vi "test_asap_coupling.vi"() -> ()   [LabVIEW 2013]
uses:
  <vilib>/Analysis/Matrix/Datatypes/RealMatrix.ctl
  <vilib>/Analysis/6fits.llb/Curve Fitting Criteria.ctl
  initialization/micron_globals.vi
  <vilib>/Analysis/Matrix/Numeric/Conversions/Array To Matrix - RA.vi
  <vilib>/Analysis/Matrix/NI_Matrix.lvlib
  <vilib>/Analysis/NI_AALPro.lvlib
panel:
  out "slope":dbl format="%#_3p"
  in  "Fit method":T1=2 items=["Least Square", "Least Absolute Residual", "Bisquare"]
  out "Error vs. sensor plane distance":cluster{cluster{sgl, "Numeric":dbl}[]}[](graph)
  out "Two-on error (axis sum, normalized)":T2 format="%#_3p"
  out "Sensor 1 1/dist":T2 format="%#_3p"
  out "Sensor 0 1/dist":T2 format="%#_3p"
  out "All-on sum":T2 format="%#_3p"
  out "Two-on error (axis sum, um)":T2 format="%#_3p"
  out "All-on axis error (um)":T2 format="%#_3p"
  out "Coupling from all lights":sgl[][](array[numeric]) format="%#_4p"
  out "Coupling (max absolute value)":T2 format="%#_3p"
  in  "Averaging time (ms)":u32=1000
  out "Coupling by channel":sgl[][][](array[numeric]) format="%#_4p"
  in  "Num lights":i32=6
  out "Testing light":i32
  out "Coupling":T2 format="%#_3p"
  # "From light"
  # "To light"
  # "Procedure:\n -- Start asap_monitor to process \"ASAP signals\"\n -- Fixture handle.  Test is done with lights fixed.\n -- Run this VI."
  # "Test light"
  # "Each column is normalized according to the channel level for the test light."
  # "To light"
  # "PSD channel"
  # "To light"
  # "PSD channel"
  # "To light"
  # "PSD axis"
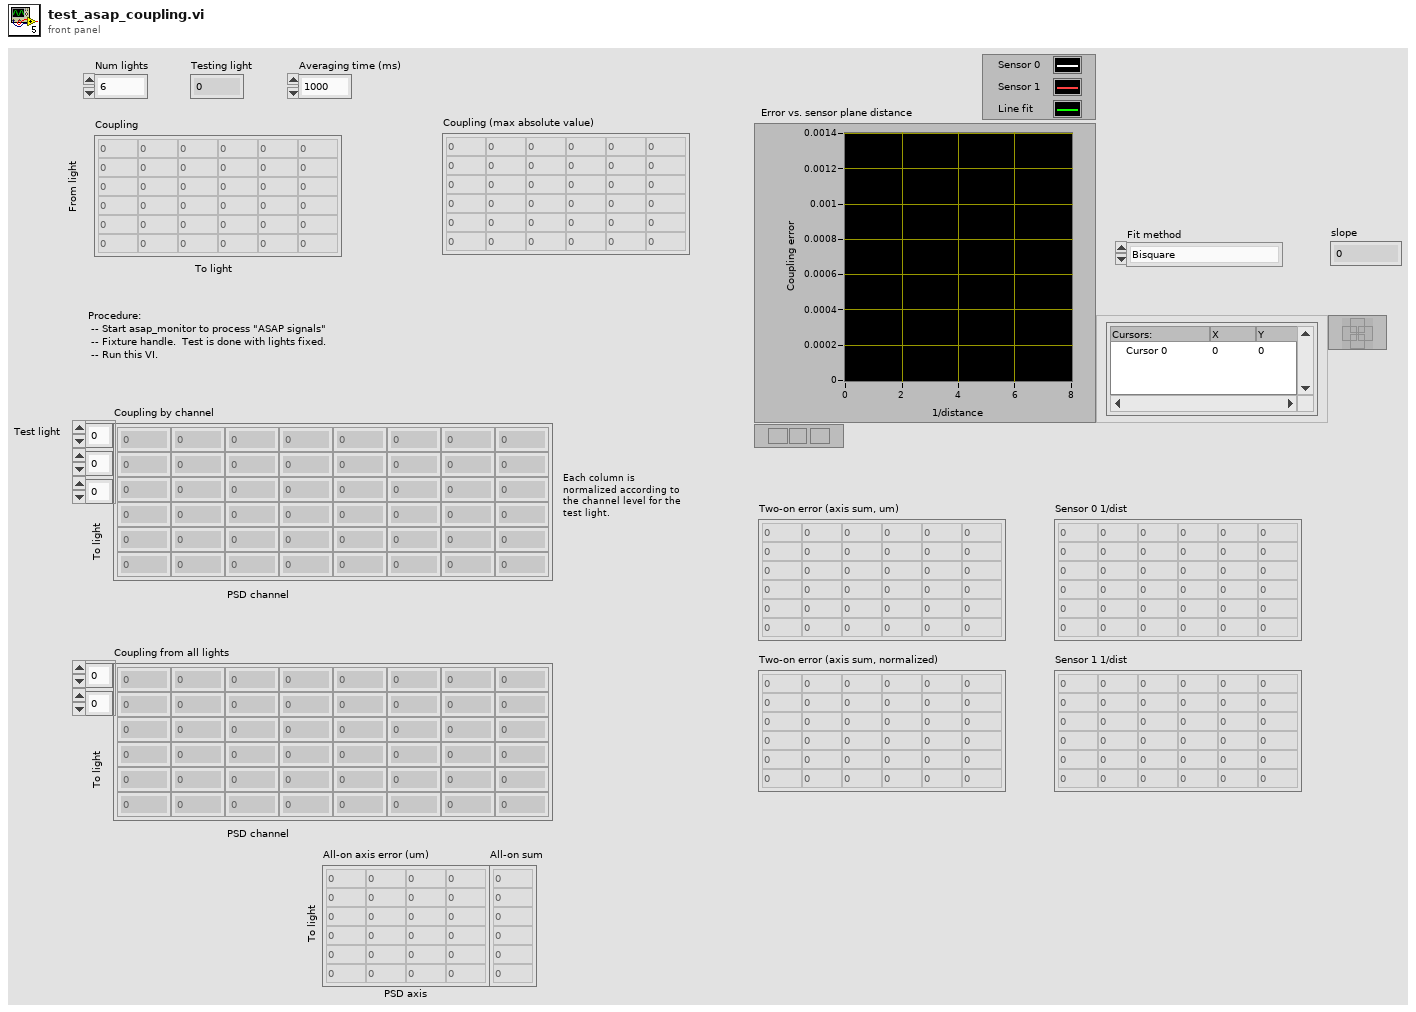
[diagram p1: front panel]
types:
  T1 = typedef "NI_AALPro.lvlib/Curve Fitting Criteria.ctl" = u16
  T2 = typedef "NI_Matrix.lvlib/RealMatrix.ctl" = dbl[][]
  T3 = typedef "micron_config.ctl" = cluster{"rt fifo":refnum<k33>, "Analog output task":refnum<k21>, "Analog output task 2":refnum<k21>, "Stimulus AO task":refnum<k21>, "Low-rate AIN task":refnum<k21>, "Pedal out task":refnum<k21>, "Pedal in task":refnum<k21>, "Loop timing source":string, "Relay out task":refnum<k21>, "Send UDP Conn":refnum<k16>, "Recv UDP Conn":refnum<k16>, "Host Addr":dbl, "I2C interface":T4, "trace_start notifier":refnum<notifier>, "trace_done notifier":refnum<notifier>, "ASAP FIFO":refnum<k33>}
  T4 = typedef "i2c_interface.ctl" = cluster{"FPGA VI Reference":T5}
  T5 = typedef "fpga_reference.ctl" = refnum<k20>
  T6 = cluster{i32, i32, "Axis positions":sgl[], "Axis positions":sgl[]}
  T7 = cluster{i32, i32, "Axis positions":sgl[], "Axis positions":sgl[]}[]
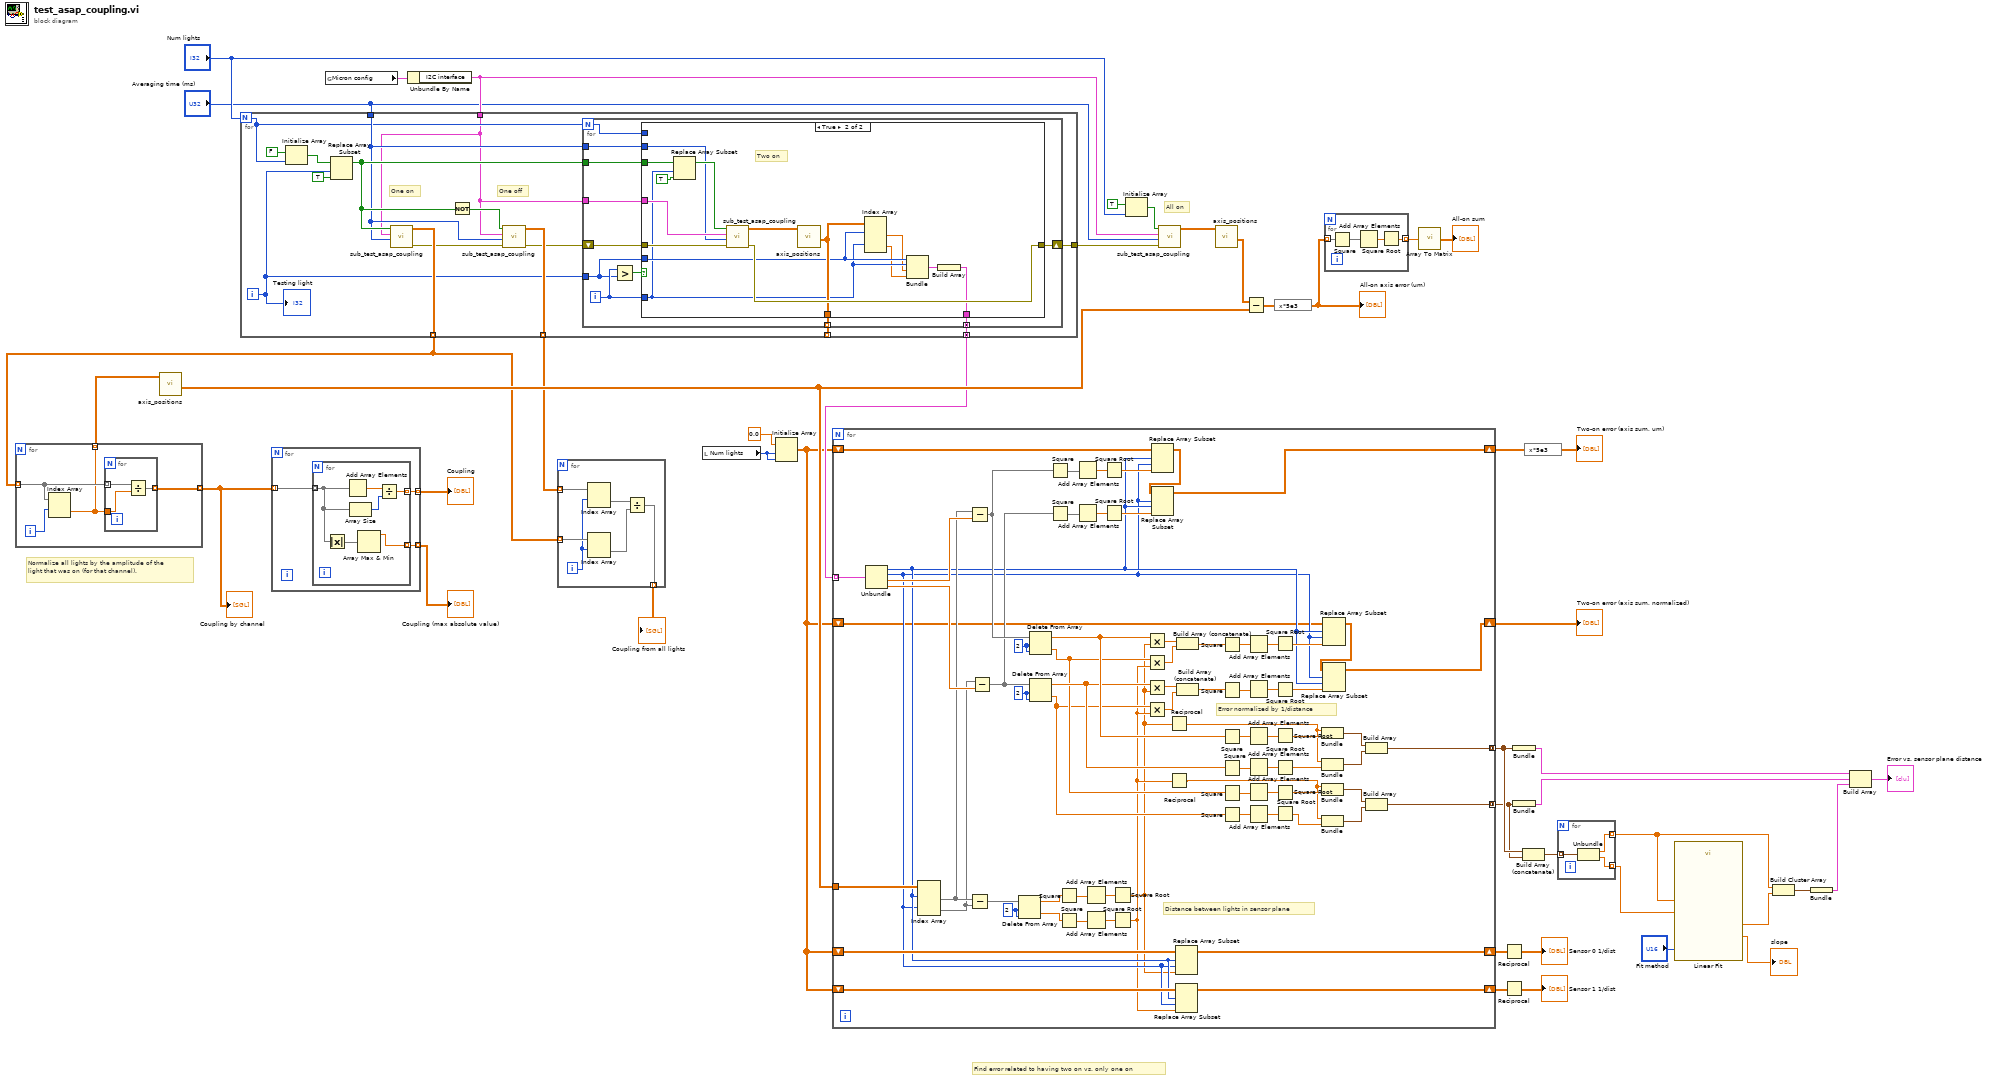
[diagram p0: block diagram]
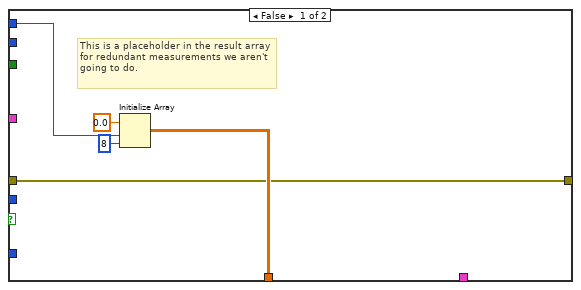
[diagram p2: hidden frame]
diagram:
  # "Find error related to having two on vs. only one on"
  # "All on"
  # "Normalize all lights by the amplitude of the light that was on (for that channel)."
  n1 = global read "micron_globals.vi" "Micron config"() -> (w42:T3)
  n2 = Unbundle By Name(w42) -> ("I2C interface"=w33:T4)
  n3 = for {
    N: "Num lights" -> [w52]
    tunnel: [w58] -> w40 mode=indexing
    tunnel: w33 -> [w47]
    tunnel: [w56] -> w39 mode=indexing
    tunnel: "Averaging time (ms)" -> [w53]
    tunnel: [w51] -> _ mode=indexing
    tunnel: [w48] -> w34
    tunnel: [w46] -> w27 mode=concatenating
    i -> [w55]
    # "One off"
    # "One on"
    n4 = Initialize Array(FALSE, w52) -> (w60:bool[])
    n5 = Replace Array Subset(array=w60, new element=TRUE ("new element/subarray"), index=w55) -> (w54:bool[])
    n6 = call "sub_test_asap_coupling.vi"("Averaging time (ms)"=w53, "I2C interface"=w47, "Light enables"=w54) -> ("error out"=w50:errorcluster, "Demodulated signals"=w58:sgl[][])  [unwired: 7 in]
    n7 = Not(x=w54) -> (.not. x?=w57:bool[])
    n8 = call "sub_test_asap_coupling.vi"("error in"=w50, "Averaging time (ms)"=w53, "I2C interface"=w47, "Light enables"=w57) -> ("error out"=w49:errorcluster, "Demodulated signals"=w56:sgl[][])  [unwired: 6 in]
    n9 = for {
      N: w52 -> [w66]
      tunnel: w55 -> [w63]
      tunnel: w54 -> [w71]
      tunnel: w47 -> [w70]
      tunnel: w53 -> [w69]
      tunnel: [w67] -> w51 mode=indexing
      shift-right: [w64] -> w48
      shift-left: w49 -> [w65]
      tunnel: [w62] -> w46 mode=concatenating
      i -> [w68]
      n10 = Greater?(x=w68, y=w63) -> (0:w72:bool)
      n11 = case shown="True" w72 {
        tunnel: w71 -> [_ w91]
        tunnel: w68 -> [_ w82]
        tunnel: w70 -> [_ w89]
        tunnel: w69 -> [_ w88]
        tunnel: [w74 w84] -> w67
        tunnel: w66 -> [w76 _]
        tunnel: w65 -> [w73 w87]
        tunnel: [w73 w86] -> w64
        tunnel: w63 -> [_ w83]
        tunnel: [_ w78] -> w62
        frame False {
          # "This is a placeholder in the result array for redundant measurements we aren't going to do."
          n12 = Initialize Array(sgl 0.0, w76, 8 ("dimension size")) -> (w74:sgl[][])
        }
        frame True {
          # "Two on"
          n13 = Replace Array Subset(array=w91, new element=TRUE ("new element/subarray"), index=w82) -> (w90:bool[])
          n14 = call "sub_test_asap_coupling.vi"("error in"=w87, "Averaging time (ms)"=w88, "I2C interface"=w89, "Light enables"=w90) -> ("error out"=w86:errorcluster, "Demodulated signals"=w85:sgl[][])  [unwired: 6 in]
          n15 = call "axis_positions.vi"("Demodulated signals"=w85) -> ("Axis positions"=w84:sgl[][])  [unwired: 8 in, 2 out]
          n16 = Index Array(array=w84, index (row) #1=w83, index (row) #2=w82) -> (element #1=w81:sgl[], element #2=w80:sgl[])  [unwired: 2 in]
          n17 = Bundle(w83, w82, "Axis positions"=w81, "Axis positions"=w80) -> (w79:T6)  [unwired: 1 in]
          n18 = Build Array(w79) -> (w78:T7)
        }
      }
    }
    "Testing light" <- w55
  }
  n19 = for {
    tunnel: w40 -> [w95] mode=indexing
    tunnel: [w94] -> w44 mode=indexing
    tunnel: [w93] -> w31 mode=indexing
    i -> [w96]
    n20 = Index Array(array=w95, index (row)=w96) -> (element=w93:sgl[])  [unwired: 1 in]
    n21 = for {
      tunnel: w93 -> [w98]
      tunnel: w95 -> [w99] mode=indexing
      tunnel: [w97] -> w94 mode=indexing
      n22 = Divide(x=w99, y=w98) -> (x/y=w97:sgl[])
    }
  }
  "Coupling by channel" <- w44
  n23 = call "axis_positions.vi"("Demodulated signals"=w31) -> ("Axis positions"=w45:sgl[][])  [unwired: 8 in, 2 out]
  n24 = for {
    tunnel: w44 -> [w100] mode=indexing
    tunnel: [w102] -> w43 mode=indexing
    tunnel: [w101] -> w41 mode=indexing
    n25 = for {
      tunnel: w100 -> [w106] mode=indexing
      tunnel: [w107] -> w102 mode=indexing
      tunnel: [w103] -> w101 mode=indexing
      n26 = Absolute Value(x=w106) -> (abs(x)=w104:sgl[])
      n27 = Add Array Elements(numeric array=w106) -> (sum=w108:sgl)
      n28 = Array Size(array=w106) -> (size(s)=w105:i32)
      n29 = Array Max & Min(array=w104) -> (max value=w103:sgl)  [unwired: 3 out]
      n30 = Divide(x=w108, y=w105) -> (x/y=w107:sgl)
    }
  }
  "Coupling" <- w43
  "Coupling (max absolute value)" <- w41
  n31 = for {
    tunnel: w40 -> [w114] mode=indexing
    tunnel: [w112] -> w38 mode=indexing
    tunnel: w39 -> [w111] mode=indexing
    i -> [w109]
    n32 = Index Array(array=w111, index (row)=w109) -> (element=w110:sgl[])  [unwired: 1 in]
    n33 = Index Array(array=w114, index (row)=w109) -> (element=w113:sgl[])  [unwired: 1 in]
    n34 = Divide(x=w110, y=w113) -> (x/y=w112:sgl[])
  }
  "Coupling from all lights" <- w38
  n35 = local read "Num lights"() -> (w26:i32)
  n36 = Initialize Array(sgl 0.0, w26, w26) -> (w19:sgl[][])
  n37 = for {
    tunnel: w27 -> [w188] mode=indexing
    tunnel: w45 -> [w187]
    shift-right: [w176] -> w23
    shift-left: w19 -> [w186]
    shift-right: [w160] -> w4
    shift-left: w19 -> [w161]
    shift-right: [w159] -> w2
    shift-left: w19 -> [w158]
    shift-right: [w141] -> w18
    shift-left: w19 -> [w142]
    tunnel: [w124] -> w14 mode=concatenating
    tunnel: [w123] -> w13 mode=concatenating
    w164 = 2 ("length")
    w165 = 2 ("length")
    w172 = 2 ("length")
    # "Error normalized by 1/distance"
    # "Distance between lights in sensor plane"
    n38 = Unbundle(w188) -> (w144:i32, w143:i32, "Axis positions"=w185:sgl[], "Axis positions"=w180:sgl[])
    n39 = Index Array(array=w187, index (row) #1=w144, index (row) #2=w143) -> (element #1=w175:sgl[], element #2=w174:sgl[])  [unwired: 2 in]
    n40 = Subtract(x=w175, y=w185) -> (x-y=w163:sgl[])
    n41 = Subtract(x=w175, y=w174) -> (x-y=w173:sgl[])
    n42 = Subtract(x=w174, y=w180) -> (x-y=w162:sgl[])
    n43 = Delete From Array(array=w173, length=w172, index=w172) -> (deleted portion=w166:sgl[], array with subset deleted=w169:sgl[])
    n44 = Delete From Array(array=w163, length=w164, index=w164) -> (deleted portion=w130:sgl[], array with subset deleted=w132:sgl[])
    n45 = Delete From Array(array=w162, length=w165, index=w165) -> (deleted portion=w129:sgl[], array with subset deleted=w131:sgl[])
    n46 = Square(x=w163) -> (x^2=w183:sgl[])
    n47 = Square(x=w162) -> (x^2=w182:sgl[])
    n48 = Square(x=w169) -> (x^2=w170:sgl[])
    n49 = Square(x=w166) -> (x^2=w168:sgl[])
    n50 = Add Array Elements(numeric array=w183) -> (sum=w184:sgl)
    n51 = Add Array Elements(numeric array=w182) -> (sum=w181:sgl)
    n52 = Add Array Elements(numeric array=w170) -> (sum=w171:sgl)
    n53 = Add Array Elements(numeric array=w168) -> (sum=w167:sgl)
    n54 = Square Root(x=w184) -> (sqrt(x)=w179:sgl)
    n55 = Square Root(x=w181) -> (sqrt(x)=w178:sgl)
    n56 = Square Root(x=w171) -> (sqrt(x)=w116:sgl)
    n57 = Square Root(x=w167) -> (sqrt(x)=w117:sgl)
    n58 = Multiply(x=w132, y=w116) -> (x*y=w157:sgl[])
    n59 = Multiply(x=w130, y=w117) -> (x*y=w156:sgl[])
    n60 = Multiply(x=w131, y=w116) -> (x*y=w155:sgl[])
    n61 = Multiply(x=w129, y=w117) -> (x*y=w154:sgl[])
    n62 = Replace Array Subset(array=w186, new element=w179, index (row)=w144, index (col)=w143) -> (w177:sgl[][])
    n63 = Replace Array Subset(array=w177, new element=w178, index (row)=w143, index (col)=w144) -> (w176:sgl[][])
    n64 = Reciprocal(x=w116) -> (1/x=w115:sgl)
    n65 = Reciprocal(x=w117) -> (1/x=w118:sgl)
    n66 = Replace Array Subset(array=w161, new element=w116, index (row)=w144, index (col)=w143) -> (w160:sgl[][])
    n67 = Replace Array Subset(array=w158, new element=w117, index (row)=w144, index (col)=w143) -> (w159:sgl[][])
    n68 = Build Array (concatenate)(w157, w156) -> (w146:sgl[])
    n69 = Build Array (concatenate)(w155, w154) -> (w145:sgl[])
    n70 = Square(x=w146) -> (x^2=w148:sgl[])
    n71 = Square(x=w145) -> (x^2=w149:sgl[])
    n72 = Square(x=w132) -> (x^2=w139:sgl[])
    n73 = Square(x=w131) -> (x^2=w138:sgl[])
    n74 = Square(x=w130) -> (x^2=w135:sgl[])
    n75 = Square(x=w129) -> (x^2=w134:sgl[])
    n76 = Add Array Elements(numeric array=w148) -> (sum=w147:sgl)
    n77 = Add Array Elements(numeric array=w149) -> (sum=w150:sgl)
    n78 = Add Array Elements(numeric array=w139) -> (sum=w140:sgl)
    n79 = Add Array Elements(numeric array=w138) -> (sum=w137:sgl)
    n80 = Add Array Elements(numeric array=w135) -> (sum=w136:sgl)
    n81 = Add Array Elements(numeric array=w134) -> (sum=w133:sgl)
    n82 = Square Root(x=w147) -> (sqrt(x)=w151:sgl)
    n83 = Square Root(x=w150) -> (sqrt(x)=w152:sgl)
    n84 = Square Root(x=w140) -> (sqrt(x)=w128:sgl)
    n85 = Square Root(x=w137) -> (sqrt(x)=w127:sgl)
    n86 = Square Root(x=w136) -> (sqrt(x)=w120:sgl)
    n87 = Square Root(x=w133) -> (sqrt(x)=w119:sgl)
    n88 = Bundle(w115, w128) -> (w126:cluster{sgl, sgl})  [unwired: 1 in]
    n89 = Bundle(w115, w127) -> (w125:cluster{sgl, sgl})  [unwired: 1 in]
    n90 = Bundle(w118, w120) -> (w121:cluster{sgl, sgl})  [unwired: 1 in]
    n91 = Bundle(w118, w119) -> (w122:cluster{sgl, sgl})  [unwired: 1 in]
    n92 = Replace Array Subset(array=w142, new element=w151, index (row)=w144, index (col)=w143) -> (w153:sgl[][])
    n93 = Replace Array Subset(array=w153, new element=w152, index (row)=w143, index (col)=w144) -> (w141:sgl[][])
    n94 = Build Array(w126, w125) -> (w124:cluster{sgl, sgl}[])
    n95 = Build Array(w121, w122) -> (w123:cluster{sgl, sgl}[])
  }
  "Two-on error (axis sum, normalized)" <- w18
  n96 = Initialize Array(TRUE, "Num lights") -> (w35:bool[])
  n97 = call "sub_test_asap_coupling.vi"("error in"=w34, "Averaging time (ms)"="Averaging time (ms)", "I2C interface"=w33, "Light enables"=w35) -> ("Demodulated signals"=w30:sgl[][])  [unwired: 6 in, 1 out]
  n98 = call "axis_positions.vi"("Demodulated signals"=w30) -> ("Axis positions"=w29:sgl[][])  [unwired: 8 in, 2 out]
  n99 = Subtract(x=w29, y=w45) -> (x-y=w28:sgl[][])
  n100 = expression code="x*5e3"(w28) -> (w22:sgl[][])
  "All-on axis error (um)" <- w22
  n101 = for {
    tunnel: w22 -> [w190] mode=indexing
    tunnel: [w189] -> w21 mode=indexing
    n102 = Square(x=w190) -> (x^2=w192:sgl[])
    n103 = Add Array Elements(numeric array=w192) -> (sum=w191:sgl)
    n104 = Square Root(x=w191) -> (sqrt(x)=w189:sgl)
  }
  n105 = call-poly <vilib>:"Array To Matrix.vi"("Real 1D Array"=w21) -> ("Real Matrix (Column Vector)"=→"All-on sum":T2)
  n106 = Reciprocal(x=w4) -> (1/x=→"Sensor 0 1/dist":sgl[][])
  n107 = Reciprocal(x=w2) -> (1/x=→"Sensor 1 1/dist":sgl[][])
  n108 = Bundle(w14) -> (w17:cluster{cluster{sgl, sgl}[]})  [unwired: 1 in]
  n109 = Bundle(w13) -> (w16:cluster{cluster{sgl, sgl}[]})  [unwired: 1 in]
  n110 = Build Array (concatenate)(w14, w13) -> (w12:cluster{sgl, sgl}[])
  n111 = expression code="x*5e3"(w23) -> (→"Two-on error (axis sum, um)":sgl[][])
  n112 = for {
    tunnel: w12 -> [w195] mode=indexing
    tunnel: [w194] -> w9 mode=indexing
    tunnel: [w193] -> w10 mode=indexing
    n113 = Unbundle(w195) -> (w194:sgl, w193:sgl)
  }
  n114 = call <vilib>:"Linear Fit.vi"("Y"=w10, "X"=w9, "method"="Fit method") -> ("Best Linear Fit"=w8:dbl[], "slope"=→"slope":dbl)  [unwired: 8 in, 3 out]
  n115 = Build Cluster Array(w9, w8) -> (w6:cluster{sgl, "Numeric":dbl}[])
  n116 = Bundle(w6) -> (w5:cluster{cluster{sgl, "Numeric":dbl}[]})  [unwired: 1 in]
  n117 = Build Array(w17, w16, w5) -> (→"Error vs. sensor plane distance":cluster{cluster{sgl, "Numeric":dbl}[]}[])
